vi "UpdateDialogWithGFGValue.vi"(7 "UpdateDialogWithGFGValue_Comamnd":T1, 8 "Error In":errorcluster, 10 "Variable Name":string, 11 "Dialog Enter Generic_UICtrlRefnums":T2) -> (0 "Error Out":errorcluster)   [LabVIEW 2012]
doc: "SciScan 1.2 160622"
uses:
  Dialog Enter Generic_UICtrlRefnums.ctl
  Custom Controls and Typedefs/BOOL Enum.ctl
  Custom Controls and Typedefs/Delete Button.ctl
  UpdateDialogWithGFGValue_Command.ctl
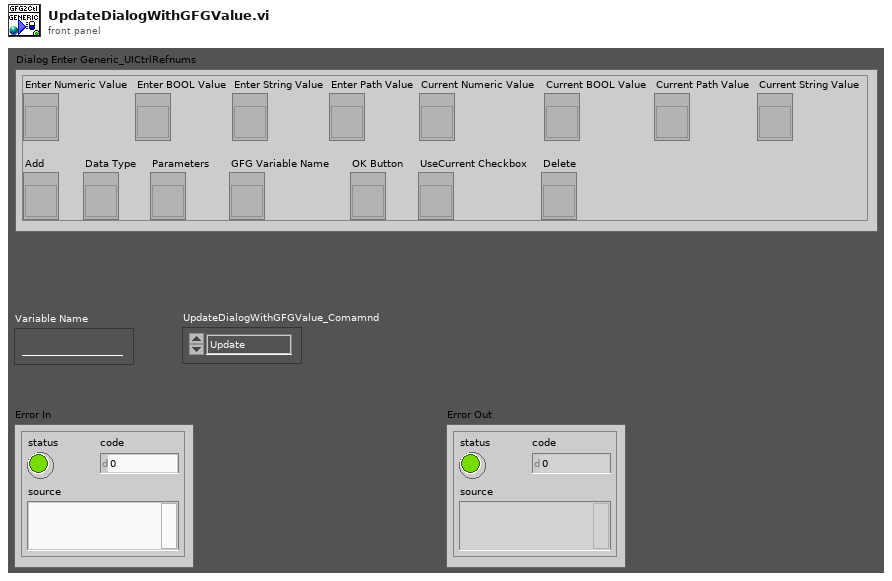
[diagram p1: front panel]
types:
  T1 = typedef "UpdateDialogWithGFGValue_Command.ctl" = enum16{"Update", "Invalidate"}
  T2 = typedef "Dialog Enter Generic_UICtrlRefnums.ctl" = cluster{"Enter Numeric Value":refnum<vi>, "Enter BOOL Value":refnum<vi>, "Enter String Value":refnum<vi>, "Enter Path Value":refnum<vi>, "Add":refnum<vi>, "Data Type":refnum<vi>, "Parameters":refnum<vi>, "GFG Variable Name":refnum<vi>, "OK Button":refnum<vi>, "Current Numeric Value":refnum<vi>, "Current BOOL Value":refnum<vi>, "Current String Value":refnum<vi>, "Current Path Value":refnum<vi>, "UseCurrent Checkbox":refnum<vi>, "Delete":refnum<vi>}
  T3 = typedef "BOOL Enum.ctl" = enum16{"FALSE", "TRUE"}
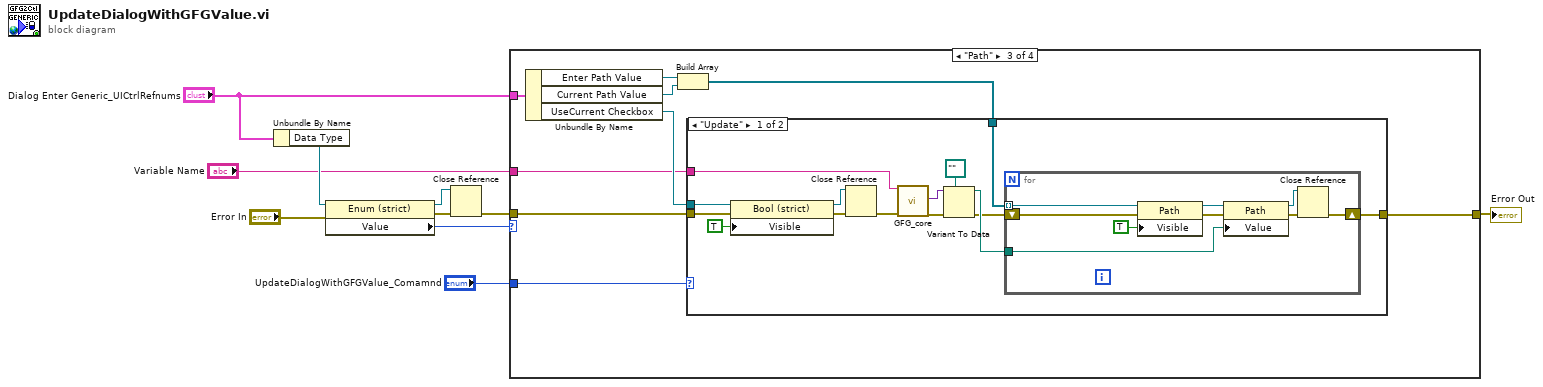
[diagram p0: block diagram]
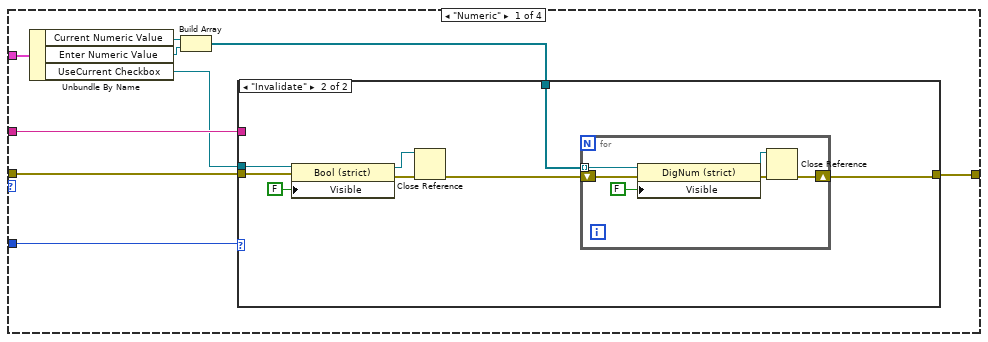
[diagram p2: hidden frame]
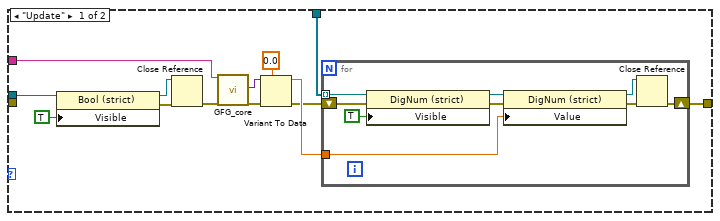
[diagram p3: hidden frame]
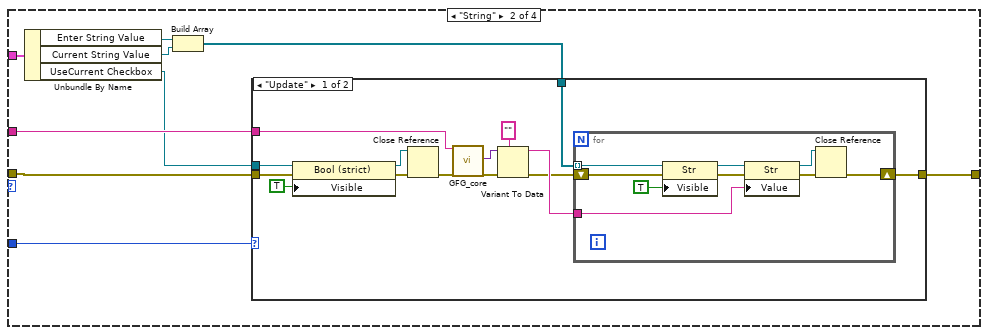
[diagram p4: hidden frame]
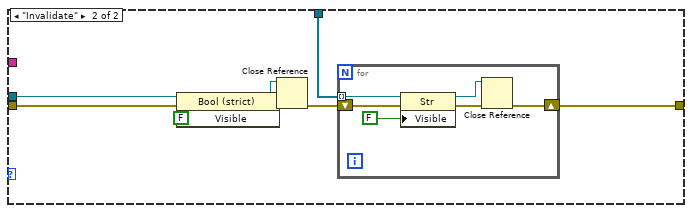
[diagram p5: hidden frame]
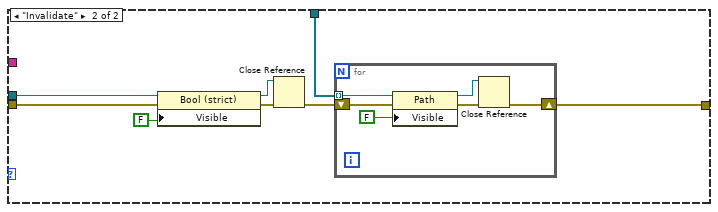
[diagram p6: hidden frame]
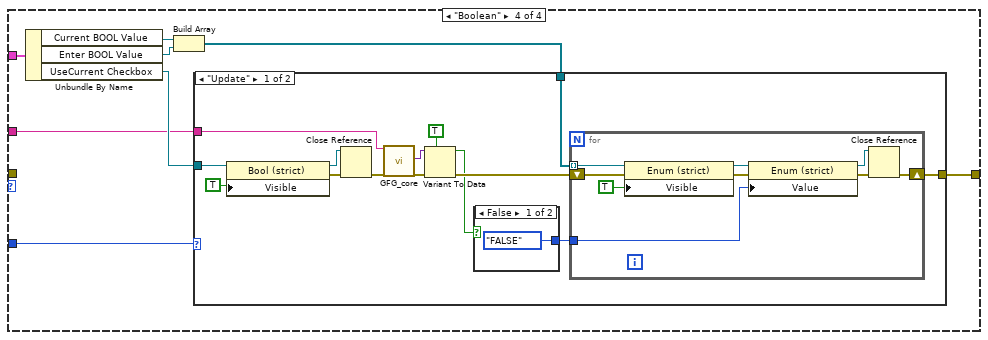
[diagram p7: hidden frame]
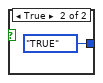
[diagram p8: hidden frame]
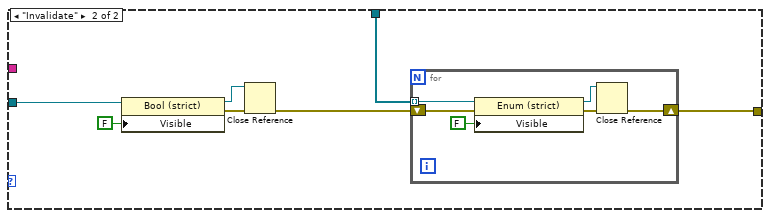
[diagram p9: hidden frame]
diagram:
  n1 = Unbundle By Name("Dialog Enter Generic_UICtrlRefnums") -> ("Data Type"=w8:refnum<vi>)
  n2 = property class="Enum (strict)"(reference=w8, error in="Error In") -> (reference out=w4:refnum<vi>, error out=w5:errorcluster, "Value"=w7:enum16{"Numeric", "Boolean", "String", "Path"})
  n3 = Close Reference(reference=w4, error in (no error)=w5) -> (error out=w1:errorcluster)
  n4 = case shown="\"Path\"" w7 {
    tunnel: "Dialog Enter Generic_UICtrlRefnums" -> [w19 w64 w110 w155]
    tunnel: [w15 w60 w106 w151] -> w6
    tunnel: "UpdateDialogWithGFGValue_Comamnd" -> [w12 w57 w104 w148]
    tunnel: "Variable Name" -> [w14 w59 w103 w149]
    tunnel: w1 -> [w11 w56 w102 _]
    frame "Numeric" {
      n5 = Unbundle By Name(w19) -> ("Current Numeric Value"=w18:refnum<vi>, "Enter Numeric Value"=w17:refnum<vi>, "UseCurrent Checkbox"=w13:refnum<vi>)
      n6 = Build Array(w18, w17) -> (w16:refnum<vi>[])
      n7 = case shown="\"Invalidate\"" w12 {
        tunnel: w16 -> [w31 w42]
        tunnel: [w28 w45] -> w15
        tunnel: w14 -> [w27 _]
        tunnel: w13 -> [w23 w44]
        tunnel: w11 -> [_ w43]
        frame "Update" {
          n8 = property class="Bool (strict)"(reference=w23, "Visible"=TRUE) -> (reference out=w21:refnum<vi>, error out=w22:errorcluster)  [unwired: 1 in]
          n9 = Close Reference(reference=w21, error in (no error)=w22) -> (error out=w20:errorcluster)
          n10 = call "GFG_core.vi"("Variable Name in"=w27, "error in (no error)"=w20) -> ("Variant Out"=w25:variant, "error out"=w26:errorcluster)  [unwired: 11 in, 5 out]
          n11 = Variant To Data(error in=w26, type=0.0, Variant=w25) -> (data=w30:dbl, error out=w29:errorcluster)
          n12 = for {
            tunnel: w31 -> [w35] mode=indexing
            tunnel: w30 -> [w41]
            shift-right: [w38] -> w28
            shift-left: w29 -> [w34]
            n13 = property class="DigNum (strict)"(reference=w35, error in=w34, "Visible"=TRUE) -> (reference out=w33:refnum<vi>, error out=w36:errorcluster)
            n14 = property class="DigNum (strict)"(reference=w33, error in=w36, "Value"=w41) -> (reference out=w39:refnum<vi>, error out=w40:errorcluster)
            n15 = Close Reference(reference=w39, error in (no error)=w40) -> (error out=w38:errorcluster)
          }
        }
        frame "Invalidate" {
          n16 = property class="Bool (strict)"(reference=w44, error in=w43, "Visible"=FALSE ("Value")) -> (reference out=w47:refnum<vi>, error out=w48:errorcluster)
          n17 = Close Reference(reference=w47, error in (no error)=w48) -> (error out=w46:errorcluster)
          n18 = for {
            tunnel: w42 -> [w55] mode=indexing
            shift-right: [w51] -> w45
            shift-left: w46 -> [w54]
            n19 = property class="DigNum (strict)"(reference=w55, error in=w54, "Visible"=FALSE) -> (reference out=w52:refnum<vi>, error out=w53:errorcluster)
            n20 = Close Reference(reference=w52, error in (no error)=w53) -> (error out=w51:errorcluster)
          }
        }
      }
    }
    frame "String" {
      n21 = Unbundle By Name(w64) -> ("Enter String Value"=w63:refnum<vi>, "Current String Value"=w62:refnum<vi>, "UseCurrent Checkbox"=w58:refnum<vi>)
      n22 = Build Array(w63, w62) -> (w61:refnum<vi>[])
      n23 = case shown="\"Update\"" w57 {
        tunnel: w61 -> [w78 w91]
        tunnel: [w75 w89] -> w60
        tunnel: w59 -> [w72 _]
        tunnel: w58 -> [w70 w90]
        tunnel: w56 -> [w65 w88]
        frame "Update" {
          n24 = property class="Bool (strict)"(reference=w70, error in=w65, "Visible"=TRUE) -> (reference out=w67:refnum<vi>, error out=w68:errorcluster)
          n25 = Close Reference(reference=w67, error in (no error)=w68) -> (error out=w66:errorcluster)
          n26 = call "GFG_core.vi"("Variable Name in"=w72, "error in (no error)"=w66) -> ("Variant Out"=w71:variant, "error out"=w73:errorcluster)  [unwired: 11 in, 5 out]
          n27 = Variant To Data(error in=w73, type="", Variant=w71) -> (data=w77:string, error out=w76:errorcluster)
          n28 = for {
            tunnel: w78 -> [w82] mode=indexing
            tunnel: w77 -> [w87]
            shift-right: [w84] -> w75
            shift-left: w76 -> [w81]
            n29 = property class="Str"(reference=w82, error in=w81, "Visible"=TRUE) -> (reference out=w79:refnum<vi>, error out=w80:errorcluster)
            n30 = property class="Str"(reference=w79, error in=w80, "Value"=w87) -> (reference out=w85:refnum<vi>, error out=w86:errorcluster)
            n31 = Close Reference(reference=w85, error in (no error)=w86) -> (error out=w84:errorcluster)
          }
        }
        frame "Invalidate" {
          n32 = property class="Bool (strict)"(reference=w90, error in=w88, "Visible"=FALSE ("Value")) -> (reference out=w93:refnum<vi>, error out=w94:errorcluster)
          n33 = Close Reference(reference=w93, error in (no error)=w94) -> (error out=w92:errorcluster)
          n34 = for {
            tunnel: w91 -> [w101] mode=indexing
            shift-right: [w97] -> w89
            shift-left: w92 -> [w100]
            n35 = property class="Str"(reference=w101, error in=w100, "Visible"=FALSE) -> (reference out=w98:refnum<vi>, error out=w99:errorcluster)
            n36 = Close Reference(reference=w98, error in (no error)=w99) -> (error out=w97:errorcluster)
          }
        }
      }
    }
    frame "Path" {
      n37 = Unbundle By Name(w110) -> ("Enter Path Value"=w109:refnum<vi>, "Current Path Value"=w108:refnum<vi>, "UseCurrent Checkbox"=w105:refnum<vi>)
      n38 = Build Array(w109, w108) -> (w107:refnum<vi>[])
      n39 = case shown="\"Update\"" w104 {
        tunnel: w107 -> [w124 w137]
        tunnel: [w121 w134] -> w106
        tunnel: w105 -> [w116 w136]
        tunnel: w103 -> [w114 _]
        tunnel: w102 -> [w113 w135]
        frame "Update" {
          n40 = property class="Bool (strict)"(reference=w116, error in=w113, "Visible"=TRUE ("Value")) -> (reference out=w112:refnum<vi>, error out=w117:errorcluster)
          n41 = Close Reference(reference=w112, error in (no error)=w117) -> (error out=w111:errorcluster)
          n42 = call "GFG_core.vi"("Variable Name in"=w114, "error in (no error)"=w111) -> ("Variant Out"=w119:variant, "error out"=w118:errorcluster)  [unwired: 11 in, 5 out]
          n43 = Variant To Data(error in=w118, type=path "", Variant=w119) -> (data=w123:path, error out=w122:errorcluster)
          n44 = for {
            tunnel: w124 -> [w126] mode=indexing
            tunnel: w123 -> [w133]
            shift-right: [w130] -> w121
            shift-left: w122 -> [w127]
            n45 = property class="Path"(reference=w126, error in=w127, "Visible"=TRUE) -> (reference out=w129:refnum<vi>, error out=w128:errorcluster)
            n46 = property class="Path"(reference=w129, error in=w128, "Value"=w133) -> (reference out=w131:refnum<vi>, error out=w132:errorcluster)
            n47 = Close Reference(reference=w131, error in (no error)=w132) -> (error out=w130:errorcluster)
          }
        }
        frame "Invalidate" {
          n48 = property class="Bool (strict)"(reference=w136, error in=w135, "Visible"=FALSE ("Value")) -> (reference out=w139:refnum<vi>, error out=w140:errorcluster)
          n49 = Close Reference(reference=w139, error in (no error)=w140) -> (error out=w138:errorcluster)
          n50 = for {
            tunnel: w137 -> [w147] mode=indexing
            shift-right: [w143] -> w134
            shift-left: w138 -> [w146]
            n51 = property class="Path"(reference=w147, error in=w146, "Visible"=FALSE) -> (reference out=w144:refnum<vi>, error out=w145:errorcluster)
            n52 = Close Reference(reference=w144, error in (no error)=w145) -> (error out=w143:errorcluster)
          }
        }
      }
    }
    frame "Boolean" {
      n53 = Unbundle By Name(w155) -> ("Current BOOL Value"=w154:refnum<vi>, "Enter BOOL Value"=w153:refnum<vi>, "UseCurrent Checkbox"=w150:refnum<vi>)
      n54 = Build Array(w154, w153) -> (w152:refnum<vi>[])
      n55 = case shown="\"Update\"" w148 {
        tunnel: w152 -> [w169 w185]
        tunnel: [w167 w181] -> w151
        tunnel: w150 -> [w163 w187]
        tunnel: w149 -> [w157 _]
        frame "Update" {
          n56 = property class="Bool (strict)"(reference=w163, "Visible"=TRUE) -> (reference out=w160:refnum<vi>, error out=w161:errorcluster)  [unwired: 1 in]
          n57 = Close Reference(reference=w160, error in (no error)=w161) -> (error out=w158:errorcluster)
          n58 = call "GFG_core.vi"("Variable Name in"=w157, "error in (no error)"=w158) -> ("Variant Out"=w156:variant, "error out"=w159:errorcluster)  [unwired: 11 in, 5 out]
          n59 = Variant To Data(error in=w159, type=TRUE, Variant=w156) -> (data=w165:bool, error out=w168:errorcluster)
          n60 = case shown="False" w165 {
            tunnel: [BOOL_Enum."FALSE" ("BOOL Enum") BOOL_Enum."TRUE" ("BOOL Enum")] -> w164
            frame False {
            }
            frame True {
            }
          }
          n61 = for {
            tunnel: w169 -> [w175] mode=indexing
            tunnel: w164 -> [w180]
            shift-right: [w177] -> w167
            shift-left: w168 -> [w173]
            n62 = property class="Enum (strict)"(reference=w175, error in=w173, "Visible"=TRUE) -> (reference out=w172:refnum<vi>, error out=w174:errorcluster)
            n63 = property class="Enum (strict)"(reference=w172, error in=w174, "Value"=w180) -> (reference out=w178:refnum<vi>, error out=w179:errorcluster)
            n64 = Close Reference(reference=w178, error in (no error)=w179) -> (error out=w177:errorcluster)
          }
        }
        frame "Invalidate" {
          n65 = property class="Bool (strict)"(reference=w187, "Visible"=FALSE ("Value")) -> (reference out=w183:refnum<vi>, error out=w184:errorcluster)  [unwired: 1 in]
          n66 = Close Reference(reference=w183, error in (no error)=w184) -> (error out=w182:errorcluster)
          n67 = for {
            tunnel: w185 -> [w193] mode=indexing
            shift-right: [w189] -> w181
            shift-left: w182 -> [w192]
            n68 = property class="Enum (strict)"(reference=w193, error in=w192, "Visible"=FALSE) -> (reference out=w190:refnum<vi>, error out=w191:errorcluster)
            n69 = Close Reference(reference=w190, error in (no error)=w191) -> (error out=w189:errorcluster)
          }
        }
      }
    }
  }
  "Error Out" <- w6
